vi "nanomsg_getsocketopt_binary.vi"(3 "error in":errorcluster, 4 "option":i32=3, 5 "level":i32=3, 6 "socket in":refnum<class "nanomsg_socket.lvclass">) -> (0 "error out":errorcluster, 1 "value":string, 2 "socket out":refnum<class "nanomsg_socket.lvclass">)   [LabVIEW 2014, in "nanomsg.lvlib" / "nanomsg_socket.lvclass"]
doc: "Query the value of <b>option</b> for the given <b>socket</b>."
uses:
  nanomsg_socket.lvclass
  nanomsg_socket.lvclass/nanomsg_socket.ctl
  <vilib>/Utility/error.llb/Error Cluster From Error Code.vi
  nanomsg.lvlib
panel:
  out "len":u32
  # "NN"
  # "labview"
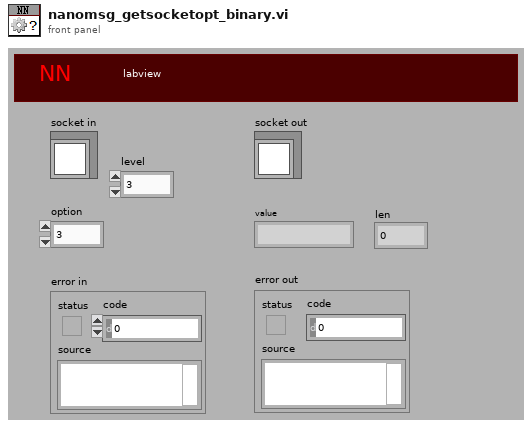
[diagram p1: front panel]
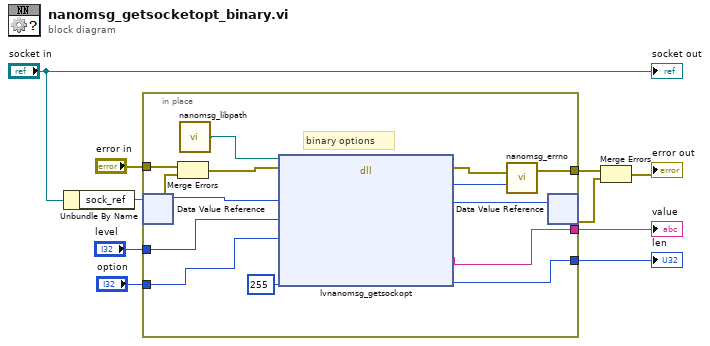
[diagram p0: block diagram]
diagram:
  n1 = Unbundle By Name("socket in") -> ("sock_ref"=w4:refnum<data-value>)
  n2 = in-place {
    in-place-border: [w22] -> w10
    in-place-border: "error in" -> [w21]
    in-place-border: "option" -> [w20]
    in-place-border: [w19] -> w7
    in-place-border: [w18] -> w6
    in-place-border: "level" -> [w12]
    # "binary options"
    n3 = in-place-dvr #1(w4) -> (w17:u64, w13:errorcluster)
    n4 = Merge Errors(w21, w13) -> (w14:errorcluster)
    n5 = call "nanomsg_libpath.vi"() -> ("path"=w15:path)
    n6 = dll-call lib="?" fn="lvnanomsg_getsockopt" ("zmq_labview.dll:lvzmq_getsockopt")(path in=w15, error in=w14, "socket"=w17, "level"=w12, "option"=w20, "len"=u32 255) -> (error out=w24:errorcluster, "return type"=w23:i32, "socket"=w16:u64, "data"=w19:string, "len"=w18:u32)  [unwired: 4 in, 1 out]
    n7 = call "nanomsg_errno.vi"("retval"=w23, "error in"=w24) -> ("error out"=w22:errorcluster)  [unwired: 1 out]
    n8 = in-place-dvr #1(w16) -> (w2:errorcluster)  [unwired: 1 out]
  }
  "value" <- w7
  "len" <- w6
  n9 = Merge Errors(w10, w2) -> (→"error out":errorcluster)
  "socket out" <- "socket in"
